vi "Set RIO INI Key.vi"(8 "error in":errorcluster, 11 "VS Engine in":refnum<class "VS Engine.lvclass">=refnum) -> (0 "error out":errorcluster, 2 "configuration file path":path, 3 "VS Engine out":refnum<class "VS Engine.lvclass">)   [LabVIEW 2024, in "VS Engine Abstraction.lvlib" / "VS Engine.lvclass"]
uses:
  VS Engine.lvclass
  VS Engine.lvclass/VS Engine.ctl
  <vilib>/NI VeriStand/Custom Device API/Custom Device API.lvlib
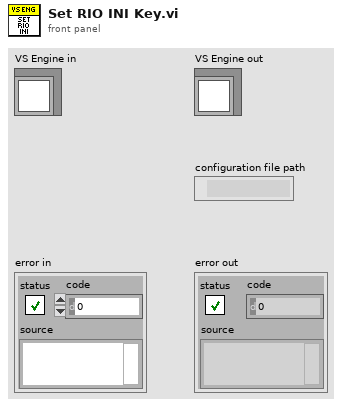
[diagram p1: front panel]
types:
  T1 = typedef "Custom Device API.lvlib/Custom Device Item Ref.ctl" = u64
  T2 = typedef "Custom Device API.lvlib/Custom Device Target Type.ctl" = enum16{"PharLap", "VxWorks", "Windows", "Linux_32_ARM", "Linux_x64"}
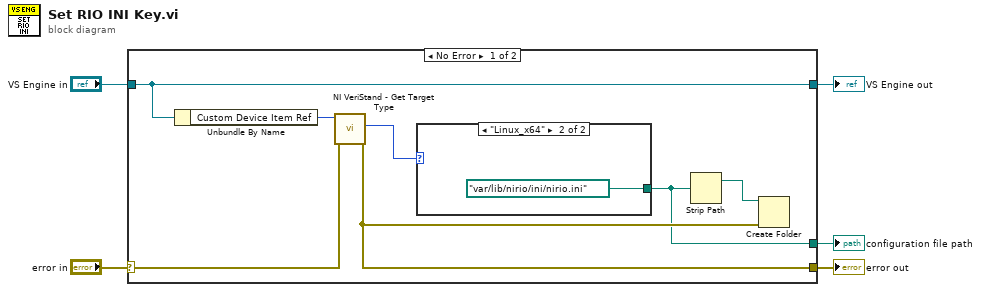
[diagram p0: block diagram]
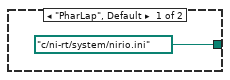
[diagram p2: hidden frame]
diagram:
  n1 = case shown="No Error" "error in" {
    selector: "error in" -> [w12 w16]
    tunnel: [w11 w16] -> w4
    tunnel: [w8 w15] -> w2
    tunnel: "VS Engine in" -> [w8 w15]
    tunnel: [w6 _] -> w1
    frame No Error {
      n2 = Unbundle By Name(w8) -> ("Custom Device Item Ref"=w7:T1)
      n3 = call <vilib>:"NI VeriStand - Get Target Type.vi"("error in (no error)"=w12, "Item Ref in"=w7) -> ("error out"=w11:errorcluster, "Target Type"=w9:T2)  [unwired: 7 in, 1 out]
      n4 = case shown="\"Linux_x64\"" w9 {
        tunnel: [path "c:/ni-rt/system/nirio.ini" ("configuration file path") path "/var/lib/nirio/ini/nirio.ini" ("configuration file path")] -> w6
        frame "PharLap", Default {
        }
        frame "Linux_x64" {
        }
      }
      n5 = Strip Path(path=w6) -> (stripped path=w10:path)  [unwired: 1 out]
      n6 = Create Folder(path (use dialog)=w10, error in=w11) -> ()  [unwired: 1 in, 3 out]
    }
    frame Error {
    }
  }
  "error out" <- w4
  "VS Engine out" <- w2
  "configuration file path" <- w1
